vi "Tempo de Processamento.vi"() -> ()   [LabVIEW 2021]
uses:
  <vilib>/numeric/Random Number (Range) U64.vi
  <vilib>/numeric/sub_Random U32.vi
panel:
  out "Tempo de Processamento":u32
  in  "upper bound (100)":u64=100
  out "# interactions":dbl
  out "Current Number":dbl
  in  "Number to match":dbl
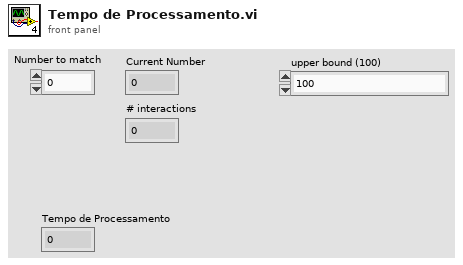
[diagram p1: front panel]
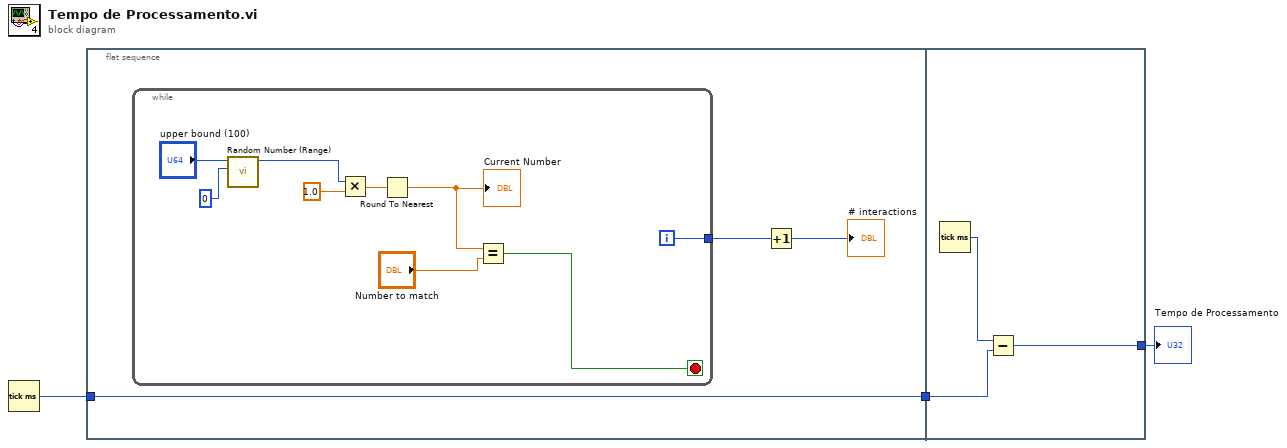
[diagram p0: block diagram]
diagram:
  n1 = Tick Count (ms)() -> (millisecond timer value=w2:u32)
  n2 = flat-sequence {
    tunnel: [w4] -> w3
    tunnel: w2 -> [w4]
    tunnel: w3 -> [w18]
    tunnel: [w16] -> w1
    frame #0 {
      n3 = while {
        tunnel: [w7] -> w6
        i -> [w7]
        stop <- w8 stop-if-true
        n4 = call-poly <vilib>:"Random Number (Range).vi"("lower bound (0)"=u64 0, "upper bound (100)"="upper bound (100)") -> ("number"=w14:u64)  [unwired: 9 in]
        n5 = Multiply(x=w14, y=1.0) -> (x*y=w13:dbl)
        n6 = Round To Nearest(number=w13) -> (nearest integer value=w9:dbl)
        "Current Number" <- w9
        n7 = Equal?(x=w9, y="Number to match") -> (x = y?=w8:bool)
      }
      n8 = Increment(x=w6) -> (x+1=→"# interactions":i32)
    }
    frame #1 {
      n9 = Tick Count (ms)() -> (millisecond timer value=w17:u32)
      n10 = Subtract(x=w17, y=w18) -> (x-y=w16:u32)
    }
  }
  "Tempo de Processamento" <- w1
